vi "Line Send Image.vi"(8 "error in":errorcluster, 10 "Image Path":path, 11 "Token":string) -> (0 "error out":errorcluster, 3 "Reply":string)   [LabVIEW 2020]
uses:
  <vilib>/httpClient/MultipartData.ctl
  <vilib>/httpClient/LabVIEWHTTPClient.lvlib
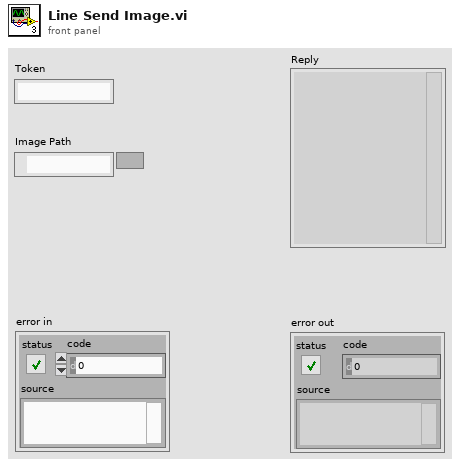
[diagram p1: front panel]
types:
  T1 = typedef "LabVIEWHTTPClient.lvlib/MultipartData.ctl" = cluster{"Name":string, "Value":string, "File":path, "Filename":string, "MIME type":string}
  T2 = typedef "LabVIEWHTTPClient.lvlib/ClientHandle.ctl" = refnum<k1>
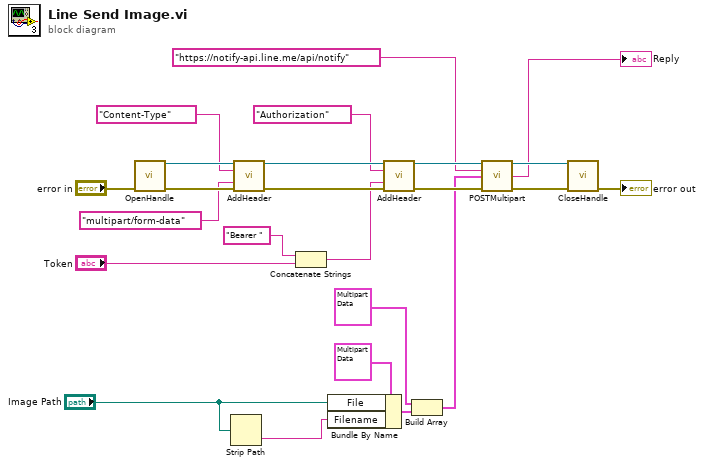
[diagram p0: block diagram]
diagram:
  n1 = call <vilib>:"OpenHandle.vi"("error in (no error)"="error in") -> ("client handle out"=w24:T2, "error out"=w23:errorcluster)  [unwired: 13 in]
  n2 = Strip Path(path="Image Path") -> (name=w2:string)  [unwired: 1 out]
  n3 = call <vilib>:"AddHeader.vi"("client handle"=w24, "header"="Content-Type", "value"="multipart/form-data", "error in (no error)"=w23) -> ("client handle out"=w20:T2, "error out"=w19:errorcluster)  [unwired: 10 in]
  n4 = Concatenate Strings("Bearer " ("string"), "Token") -> (w15:string)
  n5 = Bundle By Name(cluster=T1 {"Name"="imageFile", "Value"="", "File"=path "", "Filename"="", "MIME type"="application/octet-stream"} ("data"), "File"="Image Path", "Filename"=w2) -> (w5:T1)
  n6 = call <vilib>:"AddHeader.vi"("client handle"=w20, "header"="Authorization", "value"=w15, "error in (no error)"=w19) -> ("client handle out"=w14:T2, "error out"=w6:errorcluster)  [unwired: 10 in]
  n7 = Build Array(T1 {"Name"="message", "Value"="Send File", "File"=path "", "Filename"="", "MIME type"="application/octet-stream"} ("data"), w5) -> (w4:T1[])
  n8 = call <vilib>:"POSTMultipart.vi"("client handle"=w14, "url"="https://notify-api.line.me/api/notify", "data"=w4, "error in (no error)"=w6) -> ("client handle out"=w12:T2, "body"=→"Reply":string, "error out"=w11:errorcluster)  [unwired: 8 in, 1 out]
  n9 = call <vilib>:"CloseHandle.vi"("client handle"=w12, "error in (no error)"=w11) -> ("error out"=→"error out":errorcluster)  [unwired: 13 in]
